vi "makeClampWvfrm_v1.001.vi"(8 "# reps":i32=10, 9 "Samples to Read":i32, 10 "clamp in":T1, 11 "# Iterations":i32) -> (3 "Array":dbl[][](array[numeric]))   [LabVIEW 2019]
uses:
  Controls/clamp_profile.ctl
panel:
  out "Waveform Graph":dbl[][](graph)
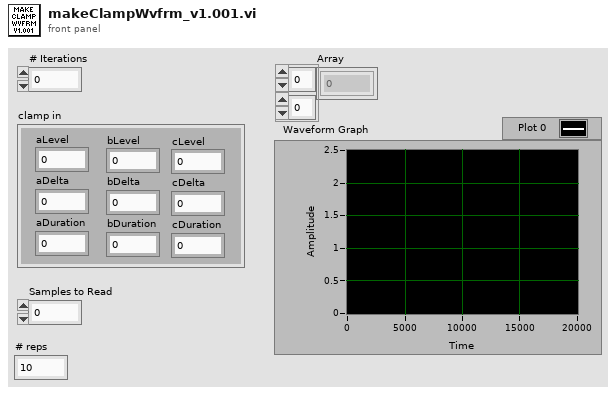
[diagram p1: front panel]
types:
  T1 = typedef "clamp_profile.ctl" = cluster{"aLevel":dbl, "aDelta":dbl, "aDuration":i32, "bLevel":dbl, "bDelta":dbl, "bDuration":i32, "cLevel":dbl, "cDelta":dbl, "cDuration":i32}
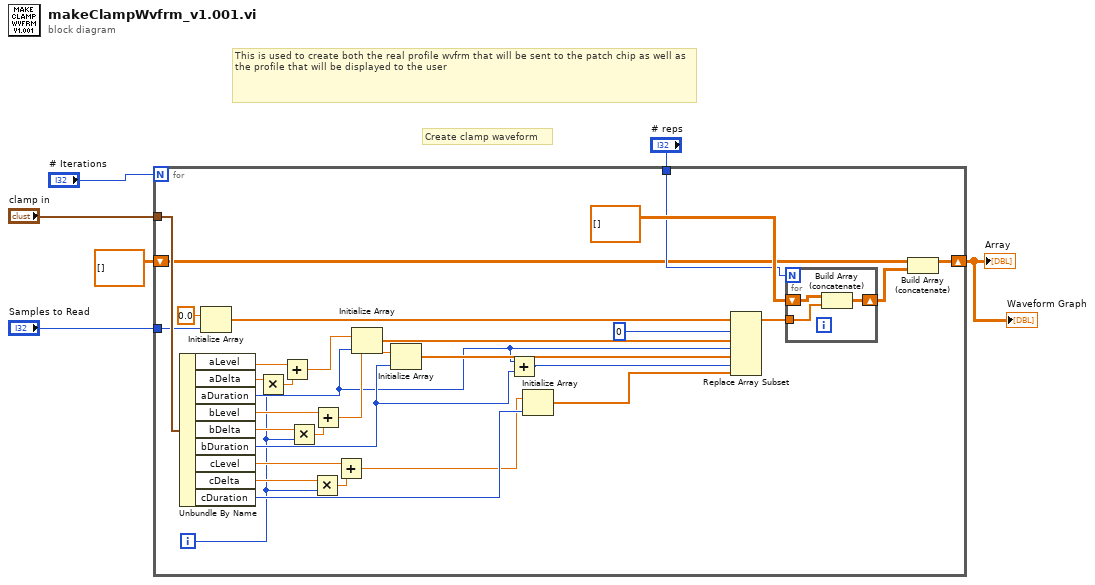
[diagram p0: block diagram]
diagram:
  # "This is used to create both the real profile wvfrm that will be sent to the patch chip as well as the profile that will be displayed to the user"
  # "Create clamp waveform"
  n1 = for {
    N: "# Iterations" -> [_]
    tunnel: "clamp in" -> [w37]
    tunnel: "Samples to Read" -> [w35]
    shift-right: [w14] -> w1
    shift-left: dbl[][] [] -> [w10]
    tunnel: "# reps" -> [w11]
    i -> [w12]
    n2 = Unbundle By Name(w37) -> ("aLevel"=w34:dbl, "aDelta"=w32:dbl, "aDuration"=w19:i32, "bLevel"=w27:dbl, "bDelta"=w26:dbl, "bDuration"=w23:i32, "cLevel"=w20:dbl, "cDelta"=w21:dbl, "cDuration"=w17:i32)
    n3 = Initialize Array(0.0, w35) -> (w15:dbl[])
    n4 = Multiply(x=w32, y=w12) -> (x*y=w33:dbl)
    n5 = Add(x=w34, y=w33) -> (x+y=w31:dbl)
    n6 = Multiply(x=w26, y=w12) -> (x*y=w29:dbl)
    n7 = Multiply(x=w21, y=w12) -> (x*y=w22:dbl)
    n8 = Add(x=w27, y=w29) -> (x+y=w28:dbl)
    n9 = Add(x=w20, y=w22) -> (x+y=w16:dbl)
    n10 = Initialize Array(w31, w19) -> (w30:dbl[])
    n11 = Initialize Array(w28, w23) -> (w25:dbl[])
    n12 = Add(x=w19, y=w23) -> (x+y=w18:i32)
    n13 = Initialize Array(w16, w17) -> (w7:dbl[])
    n14 = Replace Array Subset(array=w15, new element #1=w30, index #1=0 ("index"), new element #2=w25, index #2=w19, new element #3=w7, index #3=w18) -> (w8:dbl[])
    n15 = for {
      N: w11 -> [_]
      tunnel: w8 -> [w40]
      shift-right: [w39] -> w9
      shift-left: dbl[][] [] -> [w38]
      n16 = Build Array (concatenate)(w38, w40) -> (w39:dbl[][])
    }
    n17 = Build Array (concatenate)(w10, w9) -> (w14:dbl[][])
  }
  "Array" <- w1
  "Waveform Graph" <- w1
